vi "Inspect Configuration Tree.vi"(8 "error in (no error)":errorcluster, 11 "ConfigManager in":refnum<class "ConfigManager.lvclass">) -> (0 "error out":errorcluster, 1 "URIs":string[](array[string]), 2 "CfgManager Class Names":string[](array[string]), 3 "ConfigManager out":refnum<class "ConfigManager.lvclass">)   [LabVIEW 2013, in "CfgManager.lvlib" / "ConfigManager.lvclass"]
uses:
  ConfigManager.lvclass
  ConfigManager.lvclass/ConfigManager.ctl
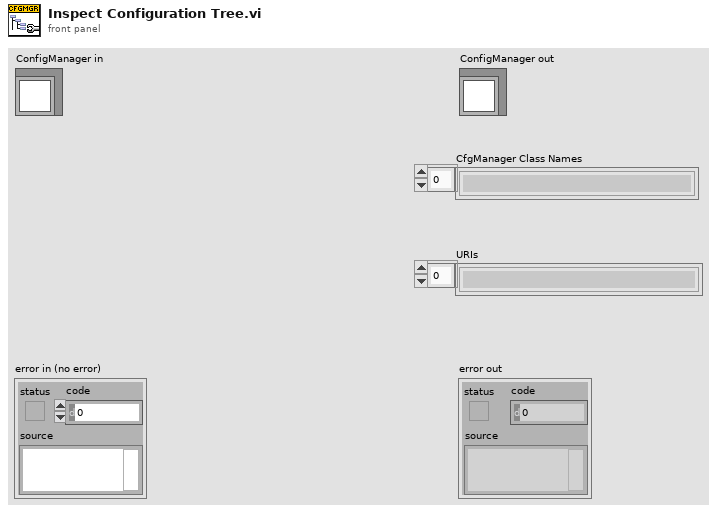
[diagram p1: front panel]
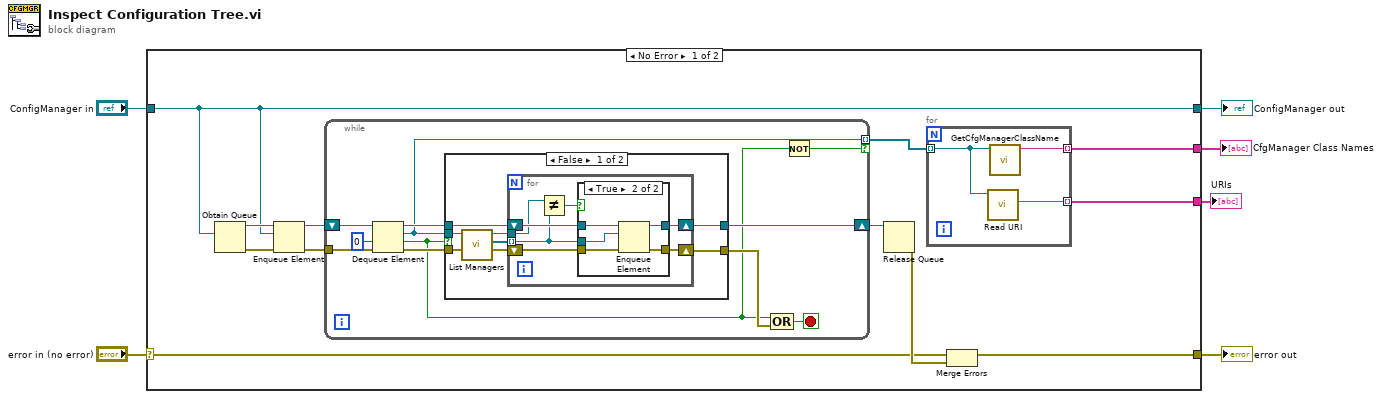
[diagram p0: block diagram]
diagram:
  n1 = case shown="No Error" "error in (no error)" {
    selector: "error in (no error)" -> [w11 w57]
    tunnel: [w10 w57] -> w5
    tunnel: [w16 w56] -> w3
    tunnel: "ConfigManager in" -> [w16 w56]
    tunnel: [w8 _] -> w2
    tunnel: [w7 _] -> w1
    frame No Error {
      n2 = Obtain Queue(element data type=w16) -> (queue out=w18:refnum<queue>, error out=w14:errorcluster)  [unwired: 4 in, 1 out]
      n3 = Enqueue Element(queue=w18, element=w16, error in (no error)=w14) -> (queue out=w17:refnum<queue>, error out=w15:errorcluster)  [unwired: 1 in, 1 out]
      n4 = while {
        tunnel: w15 -> [w29]
        shift-right: [w26] -> w13
        shift-left: w17 -> [w32]
        tunnel: [w25] -> w9 mode=indexing if=w22
        stop <- w24 stop-if-true
        n5 = Dequeue Element(queue=w32, timeout in ms (-1)=0, error in (no error)=w29) -> (queue out=w30:refnum<queue>, element=w25:refnum<class "ConfigManager.lvclass">, timed out?=w23:bool, error out=w28:errorcluster)
        n6 = case shown="False" w23 {
          tunnel: w25 -> [w39 _]
          tunnel: w30 -> [w37 w54]
          tunnel: w28 -> [w36 w55]
          tunnel: [w35 w55] -> w27
          tunnel: [w34 w54] -> w26
          frame False {
            n7 = call-dynamic "List Managers.vi"("ConfigManager in"=w39) -> ("List"=w38:refnum<class "ConfigManager.lvclass">[], "ConfigManager out"=w33:refnum<class "ConfigManager.lvclass">)  [unwired: 9 in]
            n8 = for {
              tunnel: w38 -> [w42] mode=indexing
              shift-right: [w44] -> w35
              shift-left: w36 -> [w45]
              shift-right: [w43] -> w34
              shift-left: w37 -> [w46]
              tunnel: w33 -> [w41]
              n9 = Not Equal?(x=w41, y=w42) -> (x != y?=w40:bool)
              n10 = case shown="True" w40 {
                tunnel: w46 -> [w48 w53]
                tunnel: w45 -> [w47 w52]
                tunnel: [w47 w51] -> w44
                tunnel: [w48 w50] -> w43
                tunnel: w42 -> [_ w49]
                frame False {
                }
                frame True {
                  n11 = Enqueue Element(queue=w53, element=w49, error in (no error)=w52) -> (queue out=w50:refnum<queue>, error out=w51:errorcluster)  [unwired: 1 in, 1 out]
                }
              }
            }
          }
          frame True {
          }
        }
        n12 = Compound Arithmetic op=OR(w23, w27) -> (w24:bool)
        n13 = Not(x=w23) -> (.not. x?=w22:bool)
      }
      n14 = Release Queue(queue=w13) -> (error out=w12:errorcluster)  [unwired: 2 in, 2 out]
      n15 = for {
        tunnel: w9 -> [w20] mode=indexing
        tunnel: [w21] -> w8 mode=indexing
        tunnel: [w19] -> w7 mode=indexing
        n16 = call "Read URI.vi"("ConfigManager in"=w20) -> ("URI"=w19:string)  [unwired: 9 in, 1 out]
        n17 = call "GetCfgManagerClassName.vi"("ConfigManager in"=w20) -> ("class name"=w21:string)  [unwired: 10 in]
      }
      n18 = Merge Errors(w11, w12) -> (w10:errorcluster)
    }
    frame Error {
    }
  }
  "error out" <- w5
  "ConfigManager out" <- w3
  "CfgManager Class Names" <- w2
  "URIs" <- w1
